vi "AddConsErrors.vi"(10 "Numeric":i32, 11 "Numeric 2":i32) -> (3 "Array 2":T1(array[cluster]))   [LabVIEW 2012]
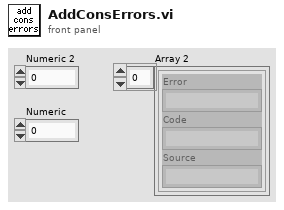
[diagram p1: front panel]
types:
  T1 = cluster{"Error":string, "Code":string, "Source":string}[]
  T2 = cluster{"Error":string, "Code":string, "Source":string}
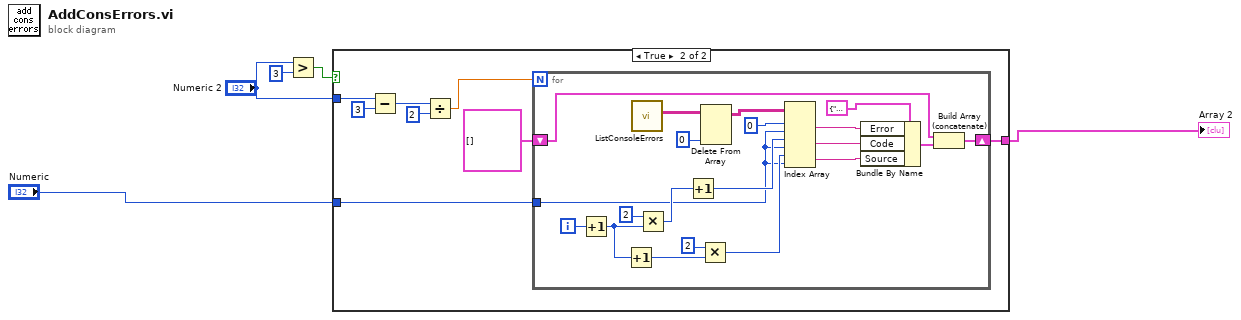
[diagram p0: block diagram]
diagram:
  n1 = Greater?(x="Numeric 2", y=3) -> (0:w1:bool)
  n2 = case shown="True" w1 {
    tunnel: "Numeric 2" -> [_ w13]
    tunnel: [_ w7] -> w5
    tunnel: "Numeric" -> [_ w6]
    frame False {
    }
    frame True {
      n3 = Subtract(x=w13, y=3) -> (x-y=w11:i32)
      n4 = Divide(x=w11, y=2) -> (x/y=w9:dbl)
      n5 = for {
        N: w9 -> [_]
        shift-right: [w30] -> w7
        shift-left: T1 [] ("Array 2") -> [w29]
        tunnel: w6 -> [w22]
        i -> [w18]
        n6 = Increment(x=w18) -> (x+1=w17:i32)
        n7 = Increment(x=w17) -> (x+1=w24:i32)
        n8 = call <userlib>:"ListConsoleErrors.vi"() -> ("Array"=w14:string[][])  [unwired: 10 in, 1 out]
        n9 = Multiply(x=2, y=w17) -> (x*y=w27:i32)
        n10 = Increment(x=w27) -> (x+1=w26:i32)
        n11 = Multiply(x=2, y=w24) -> (x*y=w23:i32)
        n12 = Delete From Array(array=w14, index (col)=0 ("disabled index (col)")) -> (array with subset deleted=w15:string[][])  [unwired: 2 in, 1 out]
        n13 = Index Array(array=w15, index (row) #1=0 ("index (row)"), index (col) #1=w22, index (row) #2=w26, index (col) #2=w22, index (row) #3=w23, index (col) #3=w22) -> (element #1=w21:string, element #2=w19:string, element #3=w20:string)
        n14 = Bundle By Name(cluster=T2 {"Error"="", "Code"="", "Source"=""} ("ConsoleError"), "Error"=w21, "Code"=w19, "Source"=w20) -> (w31:T2)
        n15 = Build Array (concatenate)(w29, w31) -> (w30:T1)
      }
    }
  }
  "Array 2" <- w5
